vi "MetaServerTCPStop.vi"(8 "error in (no error)":errorcluster) -> (0 "error out":errorcluster)   [LabVIEW 2017]
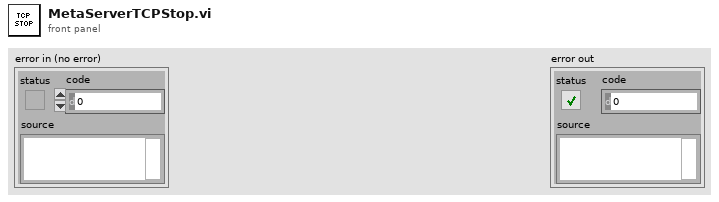
[diagram p1: front panel]
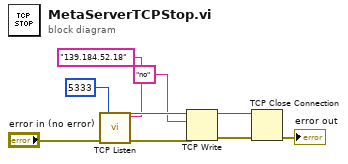
[diagram p0: block diagram]
diagram:
  n1 = call <vilib>:"TCP Listen.vi"("error in (no error)"="error in (no error)", "port"=u16 5333 ("remote port or service name"), "service name"="139.184.52.18" ("address")) -> ("error out"=w9:errorcluster, "connection ID"=w8:refnum<k5>)  [unwired: 4 in, 3 out]
  n2 = TCP Write(connection ID=w8, data in="no", error in (no error)=w9) -> (connection ID out=w6:refnum<k5>, error out=w7:errorcluster)  [unwired: 1 in, 1 out]
  n3 = TCP Close Connection(connection ID=w6, error in (no error)=w7) -> (error out=→"error out":errorcluster)  [unwired: 1 in, 1 out]
